vi "HEWH Color Check.vi"(6 "Min OK Val":dbl, 9 "Max OK Val":dbl, 10 "StDev Thresh":dbl, 11 "Panel 1":T1[](array[typedef])) -> (3 "Array":T1[](array[typedef]))   [LabVIEW 2016]
uses:
  Type Definitions/HEWH Sensor.ctl
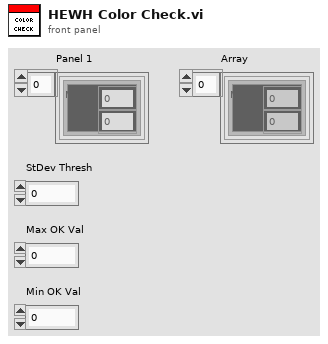
[diagram p1: front panel]
types:
  T1 = typedef "HEWH Sensor.ctl" = cluster{"Mean":dbl, " Std":dbl, "Color Box":u32}
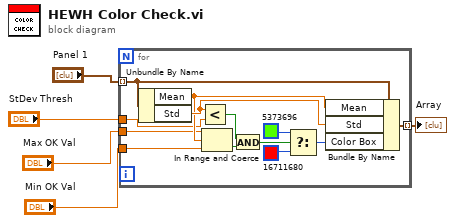
[diagram p0: block diagram]
diagram:
  n1 = for {
    tunnel: [w14] -> w1 mode=indexing
    tunnel: "Panel 1" -> [w11] mode=indexing
    tunnel: "StDev Thresh" -> [w8]
    tunnel: "Max OK Val" -> [w7]
    tunnel: "Min OK Val" -> [w6]
    n2 = Unbundle By Name(w11) -> ("Mean"=w10:dbl, "Std"=w15:dbl)
    n3 = Less?(x=w15, y=w8) -> (x < y?=w13:bool)
    n4 = In Range and Coerce(upper limit=w7, x=w10, lower limit=w6) -> (In Range?=w9:bool)  [unwired: 1 out]
    n5 = And(x=w13, y=w9) -> (x .and. y?=w12:bool)
    n6 = Select(t=u32 5373696 ("Color Box"), s=w12, f=u32 16711680 ("Color Box")) -> (s? t:f=w16:u32)
    n7 = Bundle By Name(cluster=w11, "Mean"=w10, "Std"=w15, "Color Box"=w16) -> (w14:T1)
  }
  "Array" <- w1
